vi "oa_Create Indice Reset for First No Empty Block.vi"(1 "reset in":bool, 2 "length":i32) -> (5 "reset out":bool)   [LabVIEW 2017, in "SoundVib_OAUtility.lvlib"]
uses:
  <vilib>/addons/Sound and Vibration/Order Analysis/Utility/SoundVib_OAUtility.lvlib
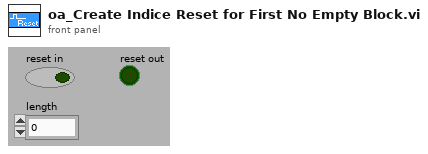
[diagram p1: front panel]
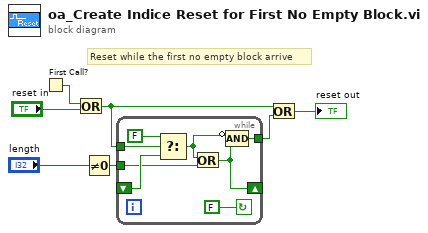
[diagram p0: block diagram]
diagram:
  # "Reset while the first no empty block arrive"
  n1 = First Call?() -> (First Call?: T/F=w7:bool)
  n2 = Or(x=w7, y="reset in") -> (x .or. y?=w3:bool)
  n3 = Not Equal To 0?(x="length") -> (x != 0?=w5:bool)
  n4 = while {
    shift-right: [w9] -> _
    shift-left: _ -> [w13]
    tunnel: w5 -> [w11]
    tunnel: w3 -> [w15]
    tunnel: [w8] -> w2
    stop <- FALSE continue-if-true
    n5 = Select(t=FALSE, s=w15, f=w13) -> (s? t:f=w10:bool)
    n6 = Or(x=w10, y=w11) -> (x .or. y?=w9:bool)
    n7 = Compound Arithmetic op=AND(invert w10, w9) -> (w8:bool)
  }
  n8 = Or(x=w3, y=w2) -> (x .or. y?=→"reset out":bool)
